vi "Test Load Snapshot - breakpoints.vi"() -> (0 "error out":errorcluster)   [LabVIEW 2020]
doc: "Test loading snapshot - only breakpoints."
uses:
  <vilib>/addons/_JKI Toolkits/Caraya/classes/Test/Test.lvclass
  src/Public API.lvlib
  src/Path Getter Mock/Path Getter Mock.lvclass
  src/Type Definitions/Snapshot Handling Options--cluster.ctl
  src/Type Definitions/Class Name--enum.ctl
  <vilib>/Utility/miscctls.llb/LVBreakpointStatusEnum.ctl
  src/Type Definitions/Breakpoint--cluster.ctl
  src/Type Definitions/Debug Snapshot--cluster.ctl
  C:/Users/juanj/Documents/hasbun_wood_engineering/github/Debug-Snapshots-for-LabVIEW/src/Path Getter Mock/Path Getter Mock.lvclass
  C:/Users/juanj/Documents/hasbun_wood_engineering/github/Debug-Snapshots-for-LabVIEW/src/IPath Getter/IPath Getter.lvclass
  <vilib>/addons/_JKI Toolkits/Caraya/classes/Assert/Assert.lvclass
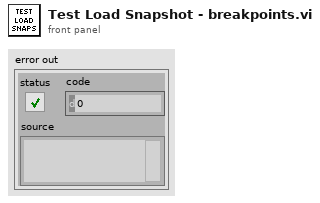
[diagram p1: front panel]
types:
  T1 = typedef "Debug Snapshot--cluster.ctl" = cluster{"VI Name":string, "Breakpoints":T2[], "Probes":i32[]}
  T2 = typedef "Breakpoint--cluster.ctl" = cluster{"UID":i32, "BP Status":T3, "Class Name":T4}
  T3 = typedef "LVBreakpointStatusEnum.ctl" = enum8{"Cleared Break", "Enabled Break", "Disabled Break"}
  T4 = typedef "Class Name--enum.ctl" = enum16{"Node", "Wire"}
  T5 = typedef "Snapshot Handling Options--cluster.ctl" = cluster{"Breakpoints":bool, "Probes":bool}
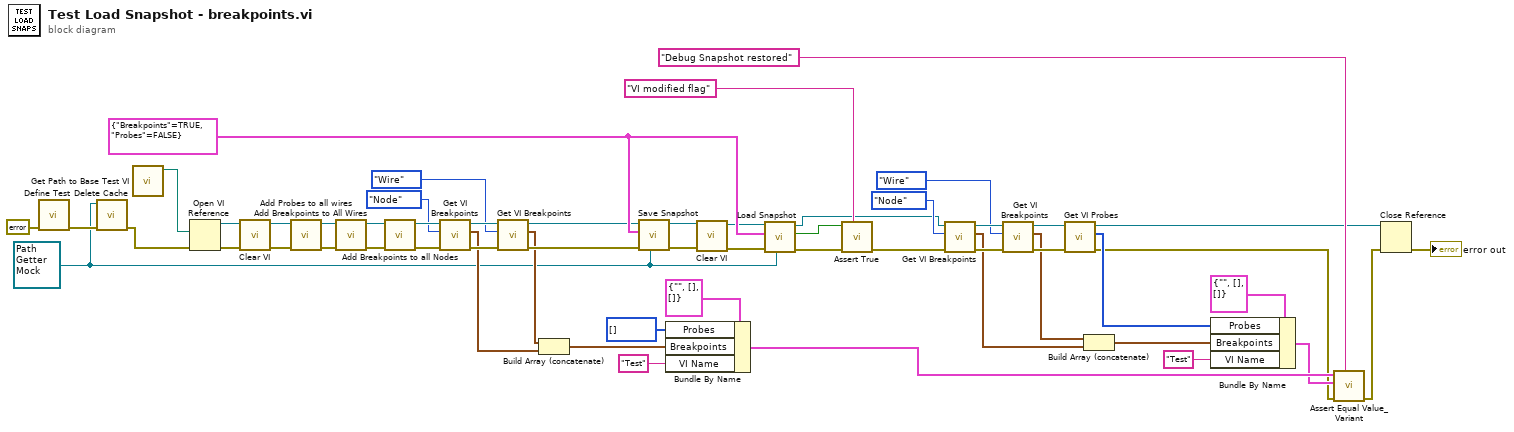
[diagram p0: block diagram]
diagram:
  w44 = T5 {"Breakpoints"=TRUE, "Probes"=FALSE} ("Debug Elements Options")
  w7 = refnum<class "Path Getter Mock.lvclass"> refnum ("Path Getter Mock.lvclass")
  n1 = call <vilib>:"Define Test.vi"("error in (no error)"=errorcluster {"status"=FALSE, "code"=0, "source"=""}) -> ("error out"=w54:errorcluster)  [unwired: 9 in, 1 out]
  n2 = call "Delete Cache.vi"("error in"=w54, "IPath Getter.lvclass"=w7) -> ("error out"=w51:errorcluster)  [unwired: 9 in]
  n3 = call "Get Path to Base Test VI.vi"() -> ("Path"=w52:path)  [unwired: 11 in]
  n4 = Open VI Reference(vi path=w52, error in (no error)=w51) -> (vi reference=w4:refnum<vi>, error out=w53:errorcluster)  [unwired: 4 in]
  n5 = call "Clear VI.vi"("error in"=w53, "VI Refnum In"=w4) -> ("error out"=w5:errorcluster, "VI Refnum Out"=w3:refnum<vi>)  [unwired: 8 in]
  n6 = call "Add Probes to all wires.vi"("error in"=w5, "VI Refnum In"=w3) -> ("error out"=w49:errorcluster, "VI Refnum Out"=w50:refnum<vi>)  [unwired: 8 in]
  n7 = call "Add Breakpoints to All Wires.vi"("error in"=w49, "VI Refnum In"=w50) -> ("error out"=w47:errorcluster, "VI Refnum Out"=w48:refnum<vi>)  [unwired: 8 in]
  n8 = call "Add Breakpoints to all Nodes.vi"("error in"=w47, "VI Refnum In"=w48) -> ("error out"=w42:errorcluster, "VI Refnum Out"=w43:refnum<vi>)  [unwired: 8 in]
  n9 = call "Get VI Breakpoints.vi"("error in"=w42, "Class Name"=Class_Name--enum."Node", "VI Reference in"=w43) -> ("error out"=w40:errorcluster, "Breakpoints"=w35:T2[], "VI Reference out"=w41:refnum<vi>)  [unwired: 6 in]
  n10 = call "Get VI Breakpoints.vi"("error in"=w40, "Class Name"=Class_Name--enum."Wire", "VI Reference in"=w41) -> ("error out"=w38:errorcluster, "Breakpoints"=w34:T2[], "VI Reference out"=w39:refnum<vi>)  [unwired: 6 in]
  n11 = Build Array (concatenate)(w34, w35) -> (w31:T2[])
  n12 = call "Save Snapshot.vi"("IPath Getter in"=w7, "error in"=w38, "Debug Elements Options"=w44, "VI Reference in"=w39) -> ("error out"=w46:errorcluster, "VI Reference out"=w2:refnum<vi>)  [unwired: 6 in]
  n13 = Bundle By Name(cluster=T1 {"VI Name"="", "Breakpoints"=[], "Probes"=[]} ("Debug Snapshot"), "Probes"=i32[] [], "Breakpoints"=w31, "VI Name"="Test") -> (w13:T1)
  n14 = call "Clear VI.vi"("error in"=w46, "VI Refnum In"=w2) -> ("error out"=w45:errorcluster, "VI Refnum Out"=w1:refnum<vi>)  [unwired: 8 in]
  n15 = call "Load Snapshot.vi"("IPath Getter in"=w7, "error in"=w45, "Debug Elements Options"=w44, "VI Reference in"=w1) -> ("error out"=w23:errorcluster, "VI Modified"=w24:bool, "VI Reference out"=w21:refnum<vi>)  [unwired: 5 in]
  n16 = call <vilib>:"Assert True.vi"("Label"="VI modified flag", "error in (no error)"=w23, "True?"=w24) -> ("error out"=w20:errorcluster)  [unwired: 7 in, 1 out]
  n17 = call "Get VI Breakpoints.vi"("error in"=w20, "Class Name"=Class_Name--enum."Node", "VI Reference in"=w21) -> ("error out"=w29:errorcluster, "Breakpoints"=w14:T2[], "VI Reference out"=w30:refnum<vi>)  [unwired: 6 in]
  n18 = call "Get VI Breakpoints.vi"("error in"=w29, "Class Name"=Class_Name--enum."Wire", "VI Reference in"=w30) -> ("error out"=w27:errorcluster, "Breakpoints"=w15:T2[], "VI Reference out"=w28:refnum<vi>)  [unwired: 6 in]
  n19 = call "Get VI Probes.vi"("error in"=w27, "VI Reference in"=w28) -> ("error out"=w10:errorcluster, "Probes"=w16:i32[], "VI Reference out"=w8:refnum<vi>)  [unwired: 7 in]
  n20 = Build Array (concatenate)(w15, w14) -> (w17:T2[])
  n21 = Bundle By Name(cluster=T1 {"VI Name"="", "Breakpoints"=[], "Probes"=[]} ("Debug Snapshot"), "Probes"=w16, "Breakpoints"=w17, "VI Name"="Test") -> (w12:T1)
  n22 = call <vilib>:"Assert Equal Value_Variant.vi"("Label"="Debug Snapshot restored", "error in (no error)"=w10, "Actual"=w12, "Expected"=w13) -> ("error out"=w9:errorcluster)  [unwired: 6 in, 1 out]
  n23 = Close Reference(reference=w8, error in (no error)=w9) -> (error out=→"error out":errorcluster)
